vi "Actor Core.vi"(8 "error in":errorcluster, 11 "Motor in":refnum<class "Motor.lvclass">) -> (0 "error out":errorcluster, 3 "Actor out":refnum<class "Actor.lvclass">)   [LabVIEW 2026, in "Motor.lvlib" / "Motor.lvclass"]
doc: "<p>(<strong>Filename</strong>: <span class=\"dnl\">Actor Framework.lvlib:Actor.lvclass:Actor Core.vi</span>)</p>\n<p>Receives messages to the actor, reacts to them, and initiates any error handling that may shut the actor down.</p>\n<p>Descendant classes may override this VI to append parallel tasks for the actor to complete while it handles messages. Overrides use the <a href=\"nihelplauncher://docs/csh?context=lvcore_glang_udclass\">Call Parent Class Method</a> node.</p>"
uses:
  Motor.lvclass
  <vilib>/ActorFramework/Actor/Actor.lvclass
  Speed Values.ctl
  Motor.lvclass/Motor.ctl
  CTI-Grove/Examples/Sourcecode/cti-drivers-lv-visa-simple/Examples/Driver/CTIPicoVISA.lvlib
panel:
  out "Speed Values":T1
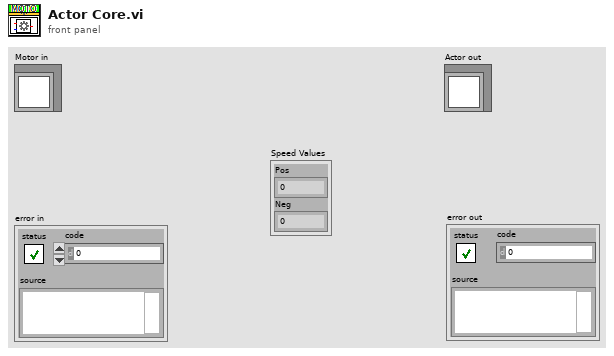
[diagram p1: front panel]
types:
  T1 = typedef "Motor.lvlib/Motor.lvclass/Speed Values.ctl" = cluster{"Pos":sgl, "Neg":sgl}
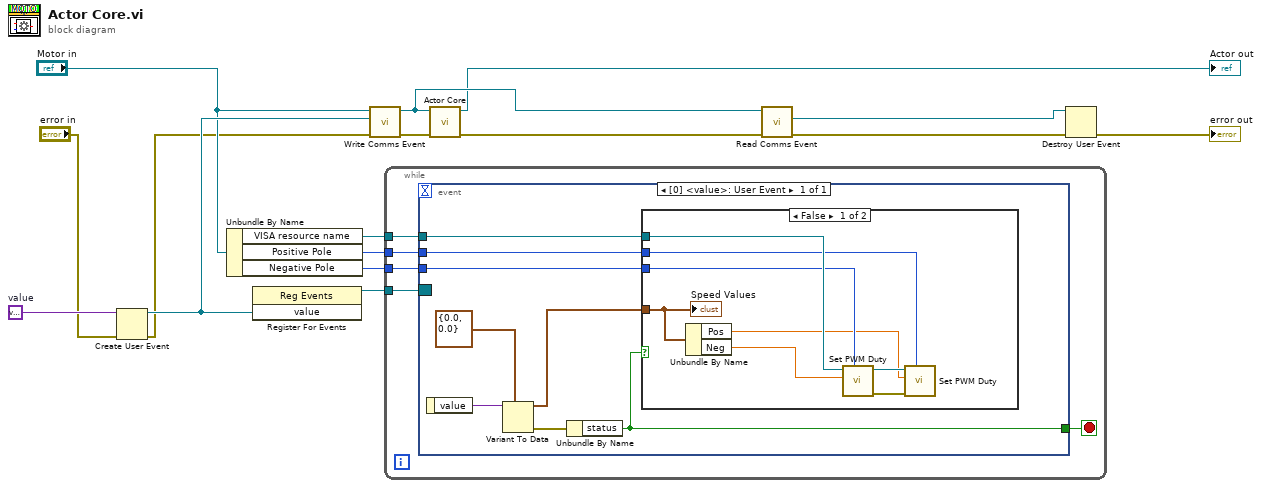
[diagram p0: block diagram]
diagram:
  w15 = variant  # value
  n1 = Create User Event(user event datatype=w15, error in="error in") -> (user event=w13:refnum<user-event>, error out=w6:errorcluster)
  n2 = Unbundle By Name("Motor in") -> ("VISA resource name"=w10:refnum<visa-resource-name>, "Positive Pole"=w9:i32, "Negative Pole"=w8:i32)
  n3 = register-events(w13) -> (reference out=w12:refnum<event-registration>)  [unwired: 2 in, 1 out]
  n4 = call-dynamic "Write Comms Event.vi"("error in (no error)"=w6, "Comms Event"=w13, "Motor in"="Motor in") -> ("error out"=w14:errorcluster, "Motor out"=w4:refnum<class "Motor.lvclass">)  [unwired: 7 in]
  n5 = while {
    tunnel: w12 -> [w21]
    tunnel: w10 -> [w19]
    tunnel: w9 -> [w18]
    tunnel: w8 -> [w17]
    stop <- w20 stop-if-true
    n6 = event shown="[0] <value>: User Event" {
      selector: w21 -> [_]
      dyn-events: _ -> [_]
      timeout: _ -> [_]
      tunnel: [w26] -> w20
      tunnel: w19 -> [w24]
      tunnel: w18 -> [w23]
      tunnel: w17 -> [w22]
      event User Event {
        n7 = event-data() -> ("value"=w29:variant)  [unwired: 1 in]
        n8 = Variant To Data(type=T1 {"Pos"=0.0, "Neg"=0.0} ("Speed Values"), Variant=w29) -> (data=w25:T1, error out=w28:errorcluster)  [unwired: 1 in]
        n9 = Unbundle By Name(w28) -> ("status"=w26:bool)
        n10 = case shown="False" w26 {
          tunnel: w25 -> [w37 _]
          tunnel: w24 -> [w36 _]
          tunnel: w23 -> [w30 _]
          tunnel: w22 -> [w35 _]
          frame False {
            n11 = Unbundle By Name(w37) -> ("Pos"=w31:sgl, "Neg"=w34:sgl)
            n12 = call "Set PWM Duty.vi"("GPIO"=w35, "Duty % (0-1)"=w34, "VISA resource name in"=w36) -> ("error out"=w32:errorcluster, "VISA resource name"=w33:refnum<visa-resource-name>)  [unwired: 7 in]
            n13 = call "Set PWM Duty.vi"("GPIO"=w30, "error in (no error)"=w32, "Duty % (0-1)"=w31, "VISA resource name in"=w33) -> ()  [unwired: 6 in, 2 out]
            "Speed Values" <- w37
          }
          frame True {
          }
        }
      }
    }
  }
  n14 = call-parent "Actor Core.vi"("error in"=w14, "Actor in"=w4) -> ("error out"=w16:errorcluster, "Actor out"=→"Actor out":refnum<class "Actor.lvclass">)  [unwired: 8 in]
  n15 = call-dynamic "Read Comms Event.vi"("error in (no error)"=w16, "Motor in"=w4) -> ("error out"=w5:errorcluster, "Comms Event"=w1:refnum<user-event>)  [unwired: 7 in, 1 out]
  n16 = Destroy User Event(user event=w1, error in=w5) -> (error out=→"error out":errorcluster)
